vi "Send Frame ID+Data Increment.vi"(5 "Data+":bool, 7 "ID+":bool, 8 "error in (no error)":errorcluster caption="错误输入（无错误）", 9 "Protocol":u32(ring)=1 items=["CAN", "CANFD"], 10 "ZCAN_TransmitFD_Data":T1, 11 "ZCAN_Transmit_Data":T2) -> (0 "error out":errorcluster caption="错误输出", 2 "ZCAN_TransmitFD_Data out":T1, 3 "ZCAN_Transmit_Data out":T2)   [LabVIEW 2011, in "CAN FD.lvlib"]
uses:
  CAN FD.lvlib
  data_type/ZCAN_Transmit_Data.ctl
  data_type/ZCAN_TransmitFD_Data.ctl
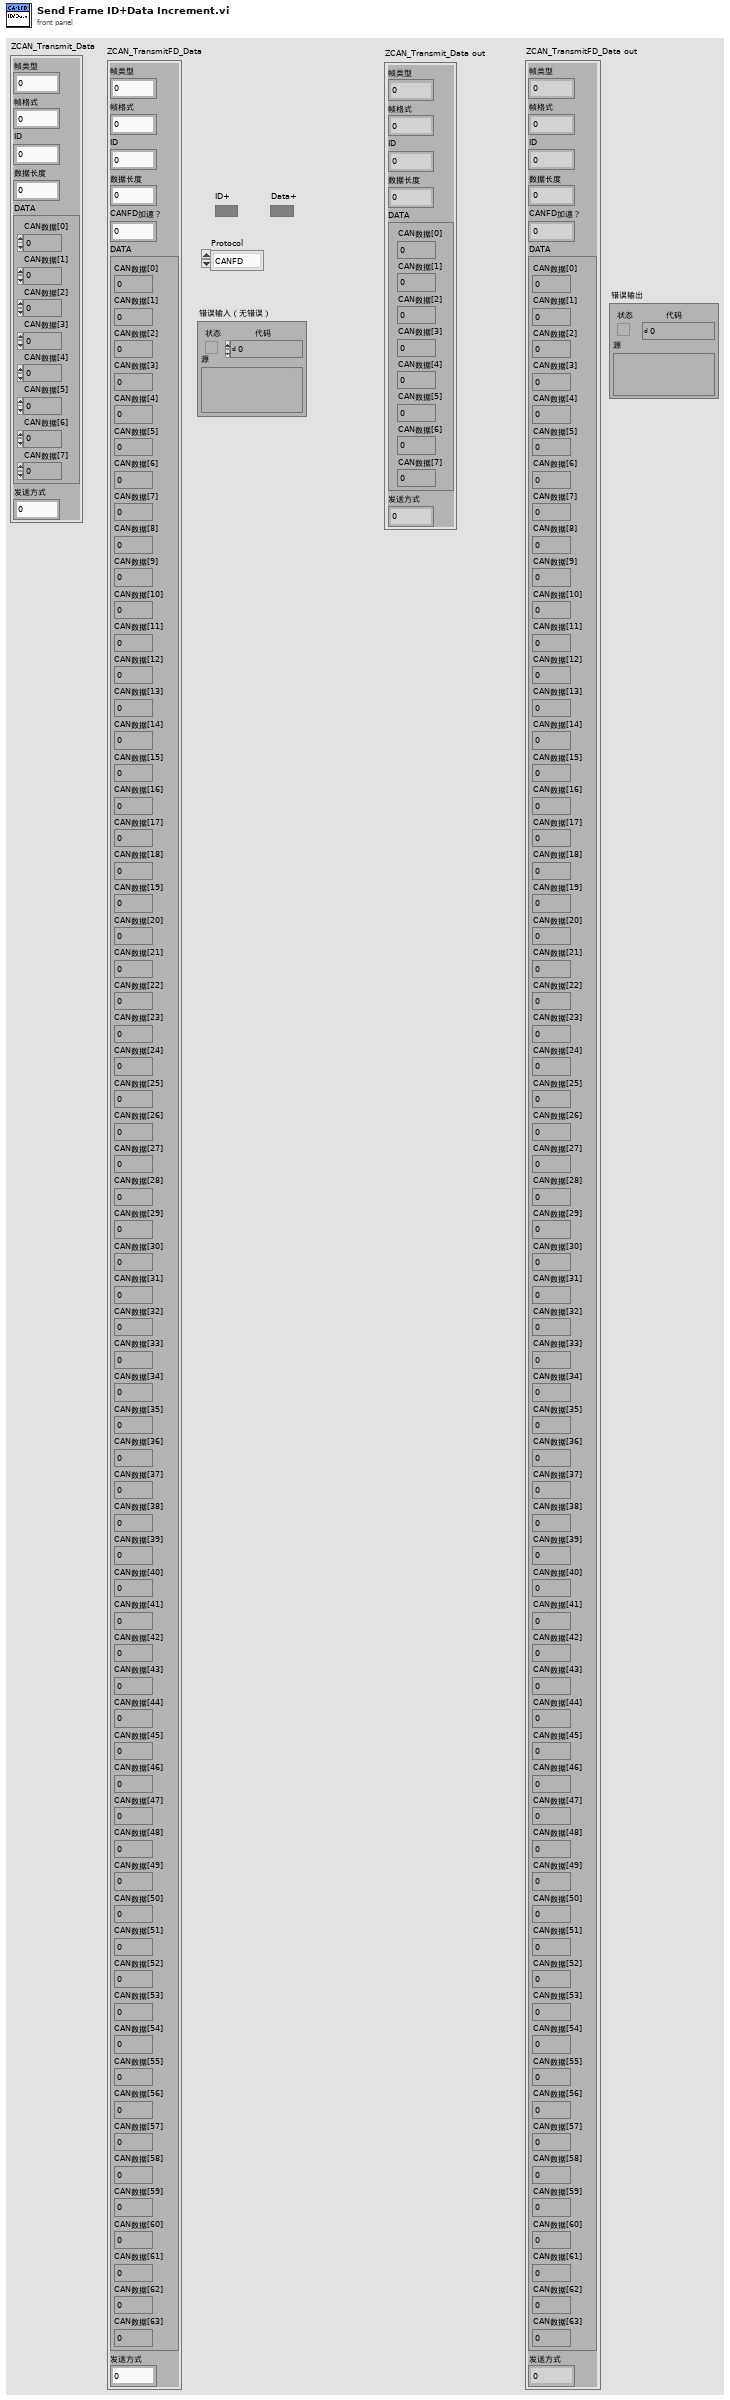
[diagram p1: front panel]
types:
  T1 = typedef "ZCAN_TransmitFD_Data.ctl" = cluster{"帧类型":u32, "帧格式":u32, "ID":u32, "数据长度":u8, "CANFD加速？":u8, "DATA":cluster{"CAN数据[0]":u8, "CAN数据[1]":u8, "CAN数据[2]":u8, "CAN数据[3]":u8, "CAN数据[4]":u8, "CAN数据[5]":u8, "CAN数据[6]":u8, "CAN数据[7]":u8, "CAN数据[8]":u8, "CAN数据[9]":u8, "CAN数据[10]":u8, "CAN数据[11] ":u8, "CAN数据[12] ":u8, "CAN数据[13] ":u8, "CAN数据[14] ":u8, "CAN数据[15] ":u8, "CAN数据[16]":u8, "CAN数据[17]":u8, "CAN数据[18]":u8, "CAN数据[19]":u8, "CAN数据[20]":u8, "CAN数据[21]":u8, "CAN数据[22]":u8, "CAN数据[23]":u8, "CAN数据[24] ":u8, "CAN数据[25]":u8, "CAN数据[26]":u8, "CAN数据[27]":u8, "CAN数据[28]":u8, "CAN数据[29]":u8, "CAN数据[30]":u8, "CAN数据[31]":u8, "CAN数据[32]":u8, "CAN数据[33]":u8, "CAN数据[34]":u8, "CAN数据[35]":u8, "CAN数据[36]":u8, "CAN数据[37]":u8, "CAN数据[38]":u8, "CAN数据[39]":u8, "CAN数据[40]":u8, "CAN数据[41]":u8, "CAN数据[42]":u8, "CAN数据[43]":u8, "CAN数据[44]":u8, "CAN数据[45]":u8, "CAN数据[46]":u8, "CAN数据[47]":u8, "CAN数据[48]":u8, "CAN数据[49]":u8, "CAN数据[50]":u8, "CAN数据[51]":u8, "CAN数据[52]":u8, "CAN数据[53]":u8, "CAN数据[54]":u8, "CAN数据[55]":u8, "CAN数据[56]":u8, "CAN数据[57]":u8, "CAN数据[58]":u8, "CAN数据[59]":u8, "CAN数据[60]":u8, "CAN数据[61]":u8, "CAN数据[62]":u8, "CAN数据[63]":u8}, "发送方式":u32}
  T2 = typedef "ZCAN_Transmit_Data.ctl" = cluster{"帧类型":u32, "帧格式":u32, "ID":u32, "数据长度":u8, "DATA":cluster{"CAN数据[0]":u8, "CAN数据[1]":u8, "CAN数据[2]":u8, "CAN数据[3]":u8, "CAN数据[4]":u8, "CAN数据[5]":u8, "CAN数据[6]":u8, "CAN数据[7]":u8}, "发送方式":u32}
  T3 = cluster{"CAN数据[0]":u8, "CAN数据[1]":u8, "CAN数据[2]":u8, "CAN数据[3]":u8, "CAN数据[4]":u8, "CAN数据[5]":u8, "CAN数据[6]":u8, "CAN数据[7]":u8}
  T4 = cluster{"Data out[0]":u8, "Data out[1]":u8, "Data out[2]":u8, "Data out[3]":u8, "Data out[4]":u8, "Data out[5]":u8, "Data out[6]":u8, "Data out[7]":u8}
  T5 = cluster{"CAN数据[0]":u8, "CAN数据[1]":u8, "CAN数据[2]":u8, "CAN数据[3]":u8, "CAN数据[4]":u8, "CAN数据[5]":u8, "CAN数据[6]":u8, "CAN数据[7]":u8, "CAN数据[8]":u8, "CAN数据[9]":u8, "CAN数据[10]":u8, "CAN数据[11] ":u8, "CAN数据[12] ":u8, "CAN数据[13] ":u8, "CAN数据[14] ":u8, "CAN数据[15] ":u8, "CAN数据[16]":u8, "CAN数据[17]":u8, "CAN数据[18]":u8, "CAN数据[19]":u8, "CAN数据[20]":u8, "CAN数据[21]":u8, "CAN数据[22]":u8, "CAN数据[23]":u8, "CAN数据[24] ":u8, "CAN数据[25]":u8, "CAN数据[26]":u8, "CAN数据[27]":u8, "CAN数据[28]":u8, "CAN数据[29]":u8, "CAN数据[30]":u8, "CAN数据[31]":u8, "CAN数据[32]":u8, "CAN数据[33]":u8, "CAN数据[34]":u8, "CAN数据[35]":u8, "CAN数据[36]":u8, "CAN数据[37]":u8, "CAN数据[38]":u8, "CAN数据[39]":u8, "CAN数据[40]":u8, "CAN数据[41]":u8, "CAN数据[42]":u8, "CAN数据[43]":u8, "CAN数据[44]":u8, "CAN数据[45]":u8, "CAN数据[46]":u8, "CAN数据[47]":u8, "CAN数据[48]":u8, "CAN数据[49]":u8, "CAN数据[50]":u8, "CAN数据[51]":u8, "CAN数据[52]":u8, "CAN数据[53]":u8, "CAN数据[54]":u8, "CAN数据[55]":u8, "CAN数据[56]":u8, "CAN数据[57]":u8, "CAN数据[58]":u8, "CAN数据[59]":u8, "CAN数据[60]":u8, "CAN数据[61]":u8, "CAN数据[62]":u8, "CAN数据[63]":u8}
  T6 = cluster{"Data out[0]":u8, "Data out[1]":u8, "Data out[2]":u8, "Data out[3]":u8, "Data out[4]":u8, "Data out[5]":u8, "Data out[6]":u8, "Data out[7]":u8, "Data out[8]":u8, "Data out[9]":u8, "Data out[10]":u8, "Data out[11]":u8, "Data out[12]":u8, "Data out[13]":u8, "Data out[14]":u8, "Data out[15]":u8, "Data out[16]":u8, "Data out[17]":u8, "Data out[18]":u8, "Data out[19]":u8, "Data out[20]":u8, "Data out[21]":u8, "Data out[22]":u8, "Data out[23]":u8, "Data out[24]":u8, "Data out[25]":u8, "Data out[26]":u8, "Data out[27]":u8, "Data out[28]":u8, "Data out[29]":u8, "Data out[30]":u8, "Data out[31]":u8, "Data out[32]":u8, "Data out[33]":u8, "Data out[34]":u8, "Data out[35]":u8, "Data out[36]":u8, "Data out[37]":u8, "Data out[38]":u8, "Data out[39]":u8, "Data out[40]":u8, "Data out[41]":u8, "Data out[42]":u8, "Data out[43]":u8, "Data out[44]":u8, "Data out[45]":u8, "Data out[46]":u8, "Data out[47]":u8, "Data out[48]":u8, "Data out[49]":u8, "Data out[50]":u8, "Data out[51]":u8, "Data out[52]":u8, "Data out[53]":u8, "Data out[54]":u8, "Data out[55]":u8, "Data out[56]":u8, "Data out[57]":u8, "Data out[58]":u8, "Data out[59]":u8, "Data out[60]":u8, "Data out[61]":u8, "Data out[62]":u8, "Data out[63]":u8}
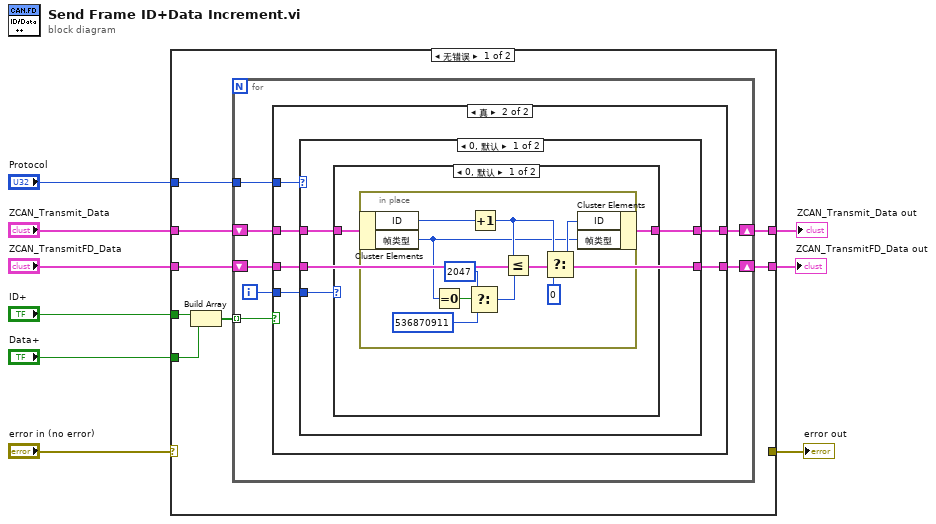
[diagram p0: block diagram]
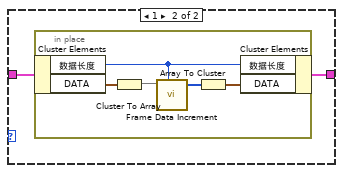
[diagram p3: hidden frame]
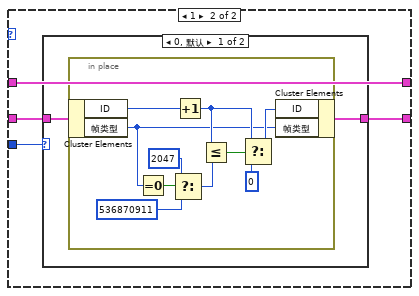
[diagram p4: hidden frame]
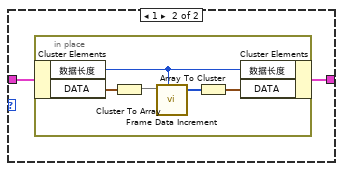
[diagram p5: hidden frame]
diagram:
  n1 = case shown="无错误" "error in (no error)" {
    selector: "error in (no error)" -> [_ w81]
    tunnel: "ID+" -> [w17 _]
    tunnel: "Data+" -> [w16 _]
    tunnel: "ZCAN_Transmit_Data" -> [w15 w80]
    tunnel: [w14 w80] -> w6
    tunnel: "Protocol" -> [w12 _]
    tunnel: "ZCAN_TransmitFD_Data" -> [w11 w79]
    tunnel: [w10 w79] -> w3
    tunnel: [_ w81] -> w1
    frame No Error {
      n2 = Build Array(w17, w16) -> (w13:bool[])
      n3 = for {
        shift-right: [w22] -> w14
        shift-left: w15 -> [w23]
        tunnel: w13 -> [w24] mode=indexing
        tunnel: w12 -> [w21]
        shift-right: [w18] -> w10
        shift-left: w11 -> [w19]
        i -> [w20]
        n4 = case shown="真" w24 {
          tunnel: w23 -> [w26 w31]
          tunnel: [w26 w29] -> w22
          tunnel: w21 -> [_ w32]
          tunnel: w20 -> [_ w30]
          tunnel: w19 -> [w25 w28]
          tunnel: [w25 w27] -> w18
          frame False {
          }
          frame True {
            n5 = case shown="0, 默认" w32 {
              tunnel: w31 -> [w35 w56]
              tunnel: w30 -> [w36 w59]
              tunnel: [w34 w56] -> w29
              tunnel: w28 -> [w33 w58]
              tunnel: [w33 w57] -> w27
              frame 0, Default {
                n6 = case shown="0, 默认" w36 {
                  tunnel: w35 -> [w38 w50]
                  tunnel: [w37 w49] -> w34
                  frame 0, Default {
                    n7 = in-place {
                      n8 = in-place-cluster #1(w38) -> ("ID"=w45:u32, "帧类型"=w43:u32)
                      n9 = Equal To 0?(x=w43) -> (x = 0?=w42:bool)
                      n10 = Select(t=u32 2047, s=w42, f=u32 536870911) -> (s? t:f=w39:u32)
                      n11 = Increment(x=w45) -> (x+1=w47:u32)
                      n12 = Less Or Equal?(x=w47, y=w39) -> (x <= y?=w48:bool)
                      n13 = Select(t=w47, s=w48, f=u32 0) -> (s? t:f=w44:u32)
                      n14 = in-place-cluster #1("ID"=w44, "帧类型"=w43) -> (w37:T2)
                    }
                  }
                  frame 1 {
                    n15 = in-place {
                      n16 = in-place-cluster #2(w50) -> ("数据长度"=w53:u8, "DATA"=w55:T3)
                      n17 = Cluster To Array(cluster=w55) -> (array=w54:u8[])
                      n18 = call "Frame Data Increment.vi"("Len"=w53, "Data in"=w54) -> ("Data out"=w52:u8[])  [unwired: 9 in]
                      n19 = Array To Cluster(array=w52) -> (cluster=w51:T4)
                      n20 = in-place-cluster #2("数据长度"=w53, "DATA"=w51) -> (w49:T2)
                    }
                  }
                }
              }
              frame 1 {
                n21 = case shown="0, 默认" w59 {
                  tunnel: w58 -> [w61 w73]
                  tunnel: [w60 w72] -> w57
                  frame 0, Default {
                    n22 = in-place {
                      n23 = in-place-cluster #3(w61) -> ("ID"=w68:u32, "帧类型"=w63:u32)
                      n24 = Equal To 0?(x=w63) -> (x = 0?=w66:bool)
                      n25 = Select(t=u32 2047, s=w66, f=u32 536870911) -> (s? t:f=w62:u32)
                      n26 = Increment(x=w68) -> (x+1=w70:u32)
                      n27 = Less Or Equal?(x=w70, y=w62) -> (x <= y?=w71:bool)
                      n28 = Select(t=w70, s=w71, f=u32 0) -> (s? t:f=w67:u32)
                      n29 = in-place-cluster #3("ID"=w67, "帧类型"=w63) -> (w60:T1)
                    }
                  }
                  frame 1 {
                    n30 = in-place {
                      n31 = in-place-cluster #4(w73) -> ("数据长度"=w76:u8, "DATA"=w78:T5)
                      n32 = Cluster To Array(cluster=w78) -> (array=w77:u8[])
                      n33 = call "Frame Data Increment.vi"("Len"=w76, "Data in"=w77) -> ("Data out"=w75:u8[])  [unwired: 9 in]
                      n34 = Array To Cluster(array=w75) -> (cluster=w74:T6)
                      n35 = in-place-cluster #4("数据长度"=w76, "DATA"=w74) -> (w72:T1)
                    }
                  }
                }
              }
            }
          }
        }
      }
    }
    frame Error {
    }
  }
  "ZCAN_Transmit_Data out" <- w6
  "ZCAN_TransmitFD_Data out" <- w3
  "error out" <- w1
